vi "validate.vi"(8 "error in":errorcluster, 11 "Standard Engine Repo Data in":refnum<class "Standard Engine Configuration.lvclass">) -> (0 "error out":errorcluster, 3 "Standard Engine Repo Data out":refnum<class "Standard Engine Configuration.lvclass">)   [LabVIEW 2013, in "Standard Engine Configuration.lvclass"]
doc: "This VI will return an error if the configuration that was input was invalid."
uses:
  Standard Engine Configuration.lvclass
  <vilib>/NI/Module Execution Interface/Engine Configuration/engine configuration.lvclass
  Standard Engine Configuration.lvclass/Standard Engine Configuration.ctl
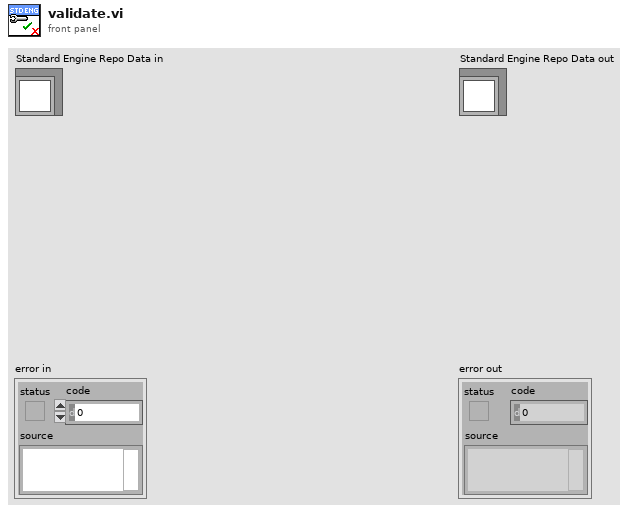
[diagram p1: front panel]
types:
  T1 = typedef "Standard Engine Configuration.lvclass/Module Specific Configuration.ctl" = cluster{"Module ID":string, "Module Decimation":T2, "error tag":string, "error responses":T3}
  T2 = typedef "Standard Engine Configuration.lvclass/Module Decimation.ctl" = cluster{"Decimation":u16, "Offset":u16, "sort order":i32, "async?":bool}
  T3 = typedef "Standard Engine Configuration.lvclass/error responses.ctl" = cluster{"unknown":T4, "trivial":T4, "critical":T4, "recoverable":T4}
  T4 = typedef "Standard Engine Configuration.lvclass/error options.ctl" = cluster{"clear":bool, "notify":bool, "remove module":bool, "abort engine":bool, "go to safe state":bool, "recover module":bool}
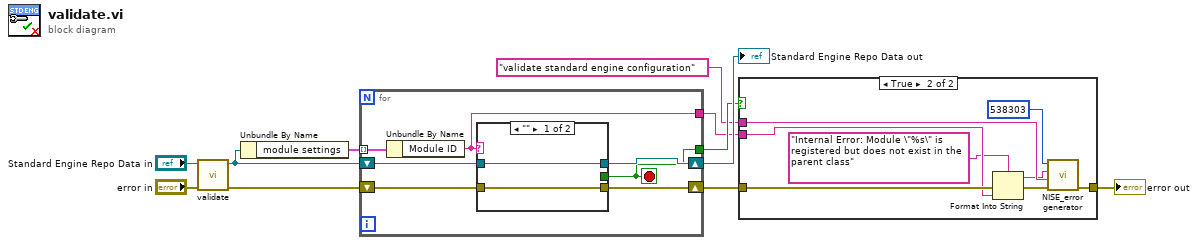
[diagram p0: block diagram]
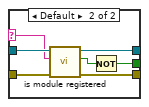
[diagram p3: hidden frame]
diagram:
  n1 = call-parent "validate.vi"("error in"="error in", "configuration in"="Standard Engine Repo Data in") -> ("error out"=w7:errorcluster, "configuration out"=w9:refnum<class "Standard Engine Configuration.lvclass">)  [unwired: 8 in]
  n2 = Unbundle By Name(w9) -> ("module settings"=w6:T1[])
  n3 = for {
    shift-right: [w18] -> w8
    shift-left: w9 -> [w17]
    shift-right: [w15] -> w2
    shift-left: w7 -> [w16]
    tunnel: w6 -> [w14] mode=indexing
    tunnel: [w12] -> w3
    tunnel: [w13] -> w4
    stop <- w13 stop-if-true
    n4 = Unbundle By Name(w14) -> ("Module ID"=w12:string)
    n5 = case shown="\"\"" w12 {
      selector: w12 -> [_ w22]
      tunnel: [w20 w27] -> w18
      tunnel: w17 -> [w20 w26]
      tunnel: w16 -> [w19 w25]
      tunnel: [w19 w24] -> w15
      tunnel: [_ w21] -> w13
      frame "" {
      }
      frame Default {
        n6 = call-dynamic "is module registered.vi"("error in"=w25, "module ID"=w22, "engine configuration in"=w26) -> ("error out"=w24:errorcluster, "registered?"=w23:bool, "engine configuration out"=w27:refnum<class "Standard Engine Configuration.lvclass">)  [unwired: 6 in]
        n7 = Not(x=w23) -> (.not. x?=w21:bool)
      }
    }
  }
  "Standard Engine Repo Data out" <- w8
  n8 = case shown="True" w4 {
    tunnel: w2 -> [w28 w36]
    tunnel: [w28 w35] -> w5
    tunnel: "validate standard engine configuration" ("source") -> [_ w33]
    tunnel: w3 -> [_ w31]
    frame False {
    }
    frame True {
      n9 = Format Into String(format string="Internal Error: Module \"%s\" is registered but does not exist in the parent class", error in=w36, w31) -> (resulting string=w29:string, error out=w32:errorcluster)  [unwired: 1 in]
      n10 = call <vilib>:"NISE_error generator.vi"("error in"=w32, "source"=w33, "append error message"=w29, "error code (0)"=538303) -> ("error out"=w35:errorcluster)  [unwired: 5 in]
    }
  }
  "error out" <- w5
